vi "Autonomous Shift Low.vi"(8 "error in (no error)":errorcluster, 11 "Solenoids In":T3) -> (0 "error out":errorcluster, 3 "Solenoids Out":T3)   [LabVIEW 2014]
uses:
  <vilib>/Rock Robotics/WPI/Solenoid/WPI_SolenoidDevRef.ctl
  <vilib>/Rock Robotics/WPI/Solenoid/WPI_SolenoidChannel.ctl
  <vilib>/Rock Robotics/WPI/Solenoid/Deprecated/WPI_SolenoidSetBool.vi
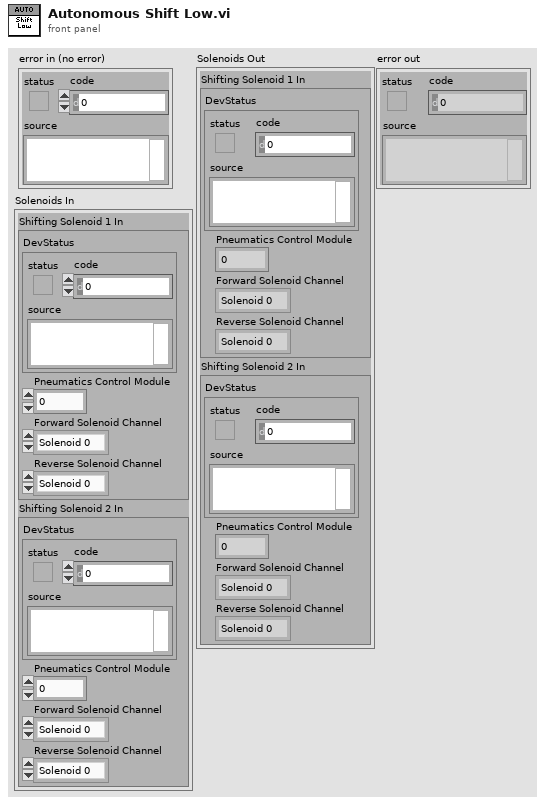
[diagram p1: front panel]
types:
  T1 = typedef "WPI_SolenoidDevRef.ctl" = cluster{"DevStatus":errorcluster, "Pneumatics Control Module":u8, "Forward Solenoid Channel":T2, "Reverse Solenoid Channel":T2}
  T2 = typedef "WPI_SolenoidChannel.ctl" = enum8{"Solenoid 0", "Solenoid 1", "Solenoid 2", "Solenoid 3", "Solenoid 4", "Solenoid 5", "Solenoid 6", "Solenoid 7", "Invalid"}
  T3 = cluster{"Shifting Solenoid 1 In":T1, "Shifting Solenoid 2 In":T1}
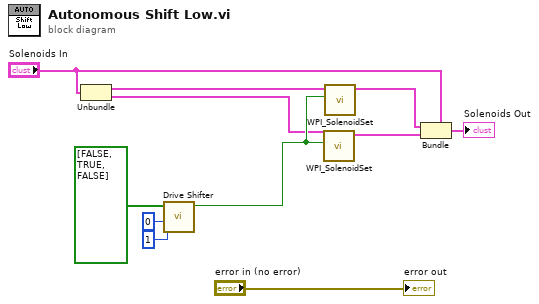
[diagram p0: block diagram]
diagram:
  n1 = Unbundle("Solenoids In") -> ("Shifting Solenoid 1 In"=w4:T1, "Shifting Solenoid 2 In"=w3:T1)
  n2 = call "Drive Shifter.vi"("Button Index Low"=1, "Button Index High"=0, "Buttons"=bool[] [FALSE, TRUE, FALSE]) -> ("High/Low"=w11:bool)  [unwired: 8 in]
  n3 = call-poly <vilib>:"WPI_SolenoidSet.vi"("Value"=w11, "SolenoidDevRef"=w3) -> ("SolenoidDevRef"=w6:T1)  [unwired: 8 in, 1 out]
  n4 = call-poly <vilib>:"WPI_SolenoidSet.vi"("Value"=w11, "SolenoidDevRef"=w4) -> ("SolenoidDevRef"=w7:T1)  [unwired: 8 in, 1 out]
  n5 = Bundle(cluster="Solenoids In", "Shifting Solenoid 1 In"=w7, "Shifting Solenoid 2 In"=w6) -> (→"Solenoids Out":T3)
  "error out" <- "error in (no error)"
